vi "subGetItemInfosFromProjectFile.vi"(8 "error in (no error)":errorcluster, 11 "SolutionBuilder in":refnum<class "SolutionBuilder.lvclass">) -> (0 "error out":errorcluster, 3 "SolutionBuilder out":refnum<class "SolutionBuilder.lvclass">)   [LabVIEW 2019, in "SolutionBuilder.lvlib" / "SolutionBuilder.lvclass"]
uses:
  SolutionBuilder.lvclass
  SolutionBuilder.lvclass/SolutionBuilder.ctl
  ProjectItem/ProjectItem.lvclass
  ProjectItem/ProjectItem.lvclass/ProjectItem.ctl
  1413a22b-f5ab-415a-875b-e08797a96725.vi
  <vilib>/xml/Load XML File.vi
  <vilib>/xml/Close Reference(Node).vi
  <vilib>/xml/NI_XML.lvlib
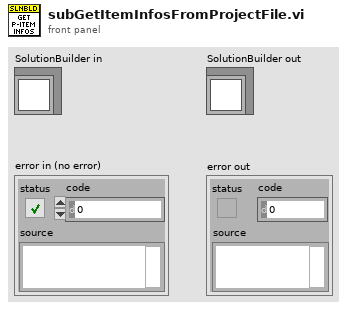
[diagram p1: front panel]
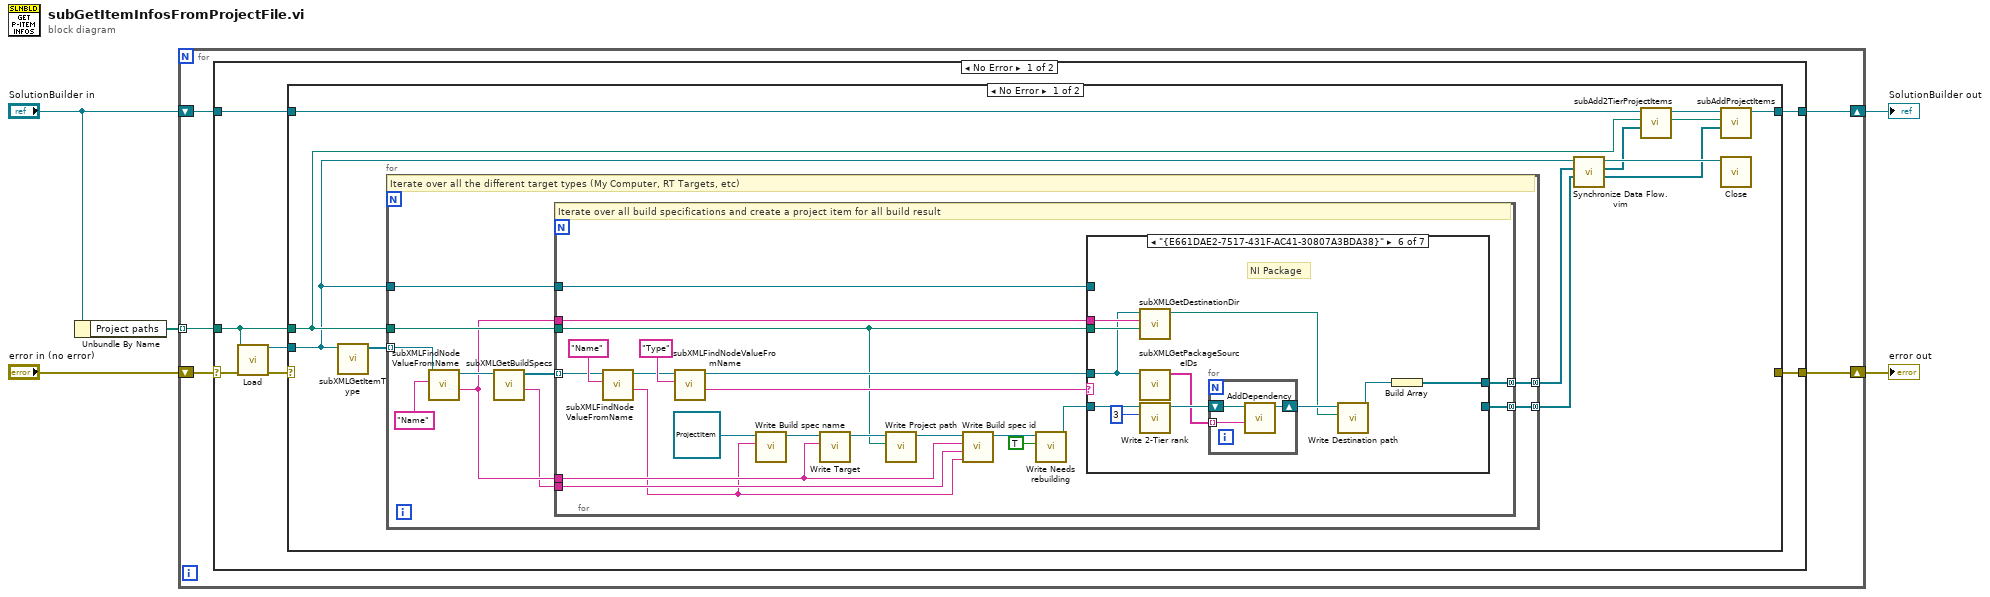
[diagram p0: block diagram]
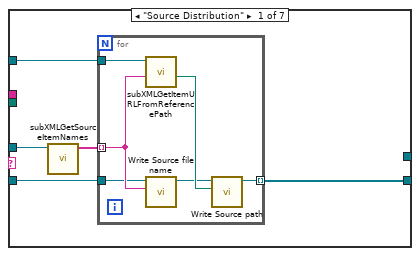
[diagram p2: hidden frame]
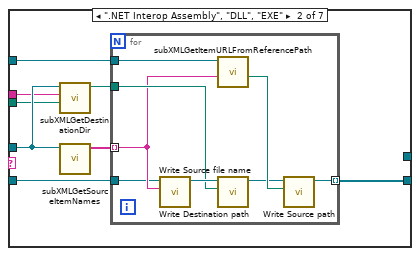
[diagram p3: hidden frame]
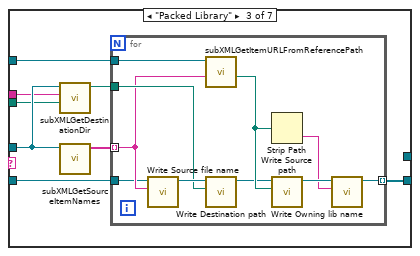
[diagram p4: hidden frame]
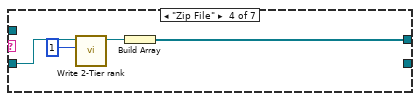
[diagram p5: hidden frame]
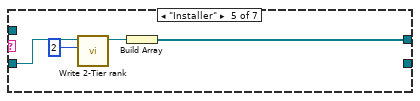
[diagram p6: hidden frame]
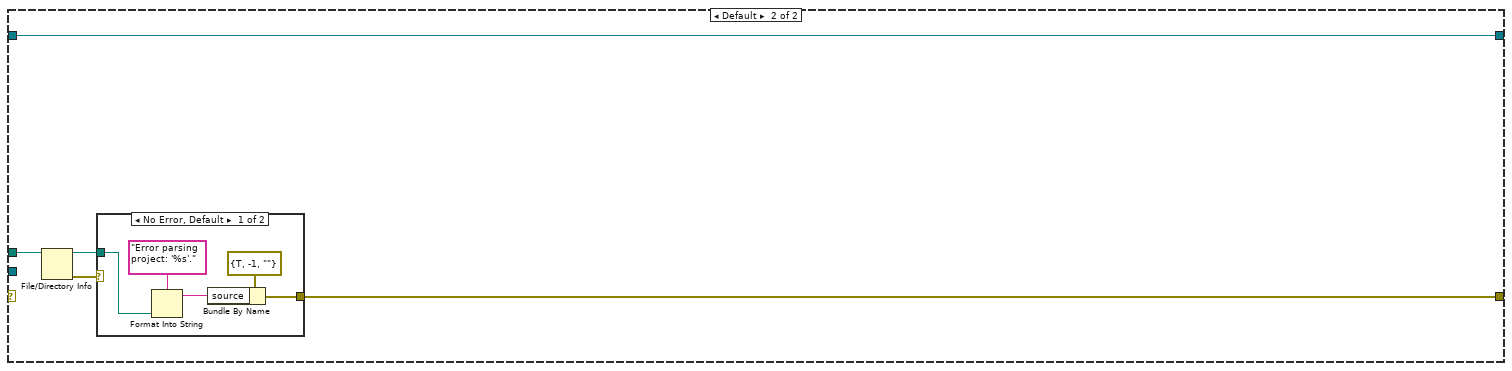
[diagram p8: hidden frame]
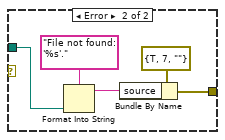
[diagram p9: hidden frame]
diagram:
  n1 = Unbundle By Name("SolutionBuilder in") -> ("Project paths"=w5:path[])
  n2 = for {
    tunnel: w5 -> [w9] mode=indexing
    shift-right: [w8] -> w3
    shift-left: "SolutionBuilder in" -> [w10]
    shift-right: [w7] -> w2
    shift-left: "error in (no error)" -> [w6]
    n3 = case shown="No Error" w6 {
      selector: w6 -> [w11 w143]
      tunnel: w10 -> [w16 w142]
      tunnel: w9 -> [w15 _]
      tunnel: [w14 w142] -> w8
      tunnel: [w12 w143] -> w7
      frame No Error {
        n4 = call-poly <vilib>:"Load.vi"("path to XML document"=w15, "error in (no error)"=w11) -> ("DOM document out"=w17:refnum<k20>, "error out"=w13:errorcluster)  [unwired: 11 in, 1 out]
        n5 = case shown="No Error" w13 {
          tunnel: w17 -> [w21 _]
          tunnel: w16 -> [w25 w131]
          tunnel: w15 -> [w23 w128]
          tunnel: [w28 w131] -> w14
          tunnel: [_ w130] -> w12
          frame No Error {
            n6 = call "subXMLGetItemType.vi"("Refnum in"=w21) -> ("Nodes"=w20:refnum<k20>[])  [unwired: 10 in]
            n7 = for {
              tunnel: [w37] -> w19 mode=concatenating
              tunnel: [w36] -> w18 mode=concatenating
              tunnel: w23 -> [w35]
              tunnel: w21 -> [w34]
              tunnel: w20 -> [w32] mode=indexing
              # "Iterate over all the different target types (My Computer, RT Targets, etc)"
              n8 = call "subXMLFindNodeValueFromName.vi"("Property name"="Name", "Refnum in"=w32) -> ("Value"=w30:string, "Refnum out"=w31:refnum<k20>)  [unwired: 7 in, 1 out]
              n9 = call "subXMLGetBuildSpecs.vi"("Refnum in"=w31) -> ("Buid spec section"=w29:string, "Nodes"=w38:refnum<k20>[])  [unwired: 9 in]
              n10 = for {
                tunnel: w38 -> [w54] mode=indexing
                tunnel: w35 -> [w44]
                tunnel: [w53] -> w37 mode=concatenating
                tunnel: w34 -> [w52]
                tunnel: [w51] -> w36 mode=concatenating
                tunnel: w30 -> [w40]
                tunnel: w30 -> [w50]
                tunnel: w29 -> [w45]
                # "Iterate over all build specifications and create a project item for all build result"
                n11 = call "subXMLFindNodeValueFromName.vi"("Property name"="Name", "Refnum in"=w54) -> ("Value"=w39:string, "Refnum out"=w55:refnum<k20>)  [unwired: 7 in, 1 out]
                n12 = call "subXMLFindNodeValueFromName.vi"("Property name"="Type", "Refnum in"=w55) -> ("Value"=w58:string, "Refnum out"=w57:refnum<k20>)  [unwired: 7 in, 1 out]
                n13 = call "Write Build spec name.vi"("Build spec name"=w39, "ProjectItem in"=refnum<class "ProjectItem.lvclass"> refnum ("SolutionBuilder.lvlib:ProjectItem.lvclass")) -> ("ProjectItem out"=w48:refnum<class "ProjectItem.lvclass">)  [unwired: 9 in]
                n14 = call "Write Target.vi"("Target"=w40, "ProjectItem in"=w48) -> ("ProjectItem out"=w49:refnum<class "ProjectItem.lvclass">)  [unwired: 9 in]
                n15 = call "Write Project path.vi"("Project path"=w44, "ProjectItem in"=w49) -> ("ProjectItem out"=w46:refnum<class "ProjectItem.lvclass">)  [unwired: 9 in]
                n16 = call-dynamic "Write Build spec id.vi"("Build spec name"=w39, "Buid spec section"=w45, "Target"=w40, "ProjectItem in"=w46) -> ("ProjectItem out"=w42:refnum<class "ProjectItem.lvclass">)  [unwired: 7 in]
                n17 = call "Write Needs rebuilding.vi"("Needs rebuilding"=TRUE, "ProjectItem in"=w42) -> ("ProjectItem out"=w41:refnum<class "ProjectItem.lvclass">)  [unwired: 9 in]
                n18 = case shown="\"{E661DAE2-7517-431F-AC41-30807A3BDA38}\"" w58 {
                  tunnel: w57 -> [w64 w76 w92 _ _ w113 _]
                  tunnel: [w62 w77 w93 _ _ _ _] -> w53
                  tunnel: w52 -> [w61 w74 w90 _ _ _ _]
                  tunnel: [_ _ _ w106 w110 w122 _] -> w51
                  tunnel: w50 -> [_ w73 w89 _ _ w118 _]
                  tunnel: w41 -> [w60 w72 w88 w105 w109 w121 _]
                  tunnel: w44 -> [_ w71 w87 _ _ w117 _]
                  frame "Source Distribution" {
                    n19 = call "subXMLGetSourceItemNames.vi"("Refnum in"=w64) -> ("Names"=w63:string[])  [unwired: 10 in]
                    n20 = for {
                      tunnel: w63 -> [w69] mode=indexing
                      tunnel: [w67] -> w62 mode=indexing
                      tunnel: w61 -> [w70]
                      tunnel: w60 -> [w65]
                      n21 = call "subXMLGetItemURLFromReferencePath.vi"("Reference path"=w69, "Root ref"=w70) -> ("Path"=w68:path)  [unwired: 7 in, 2 out]
                      n22 = call "Write Source file name.vi"("Source file name"=w69, "ProjectItem in"=w65) -> ("ProjectItem out"=w66:refnum<class "ProjectItem.lvclass">)  [unwired: 9 in]
                      n23 = call "Write Source path.vi"("Source path"=w68, "ProjectItem in"=w66) -> ("ProjectItem out"=w67:refnum<class "ProjectItem.lvclass">)  [unwired: 9 in]
                    }
                  }
                  frame ".NET Interop Assembly", "DLL", "EXE" {
                    n24 = call "subXMLGetDestinationDir.vi"("Project path"=w71, "TargetName"=w73, "Refnum in"=w76) -> ("Path"=w75:path)  [unwired: 7 in, 1 out]
                    n25 = call "subXMLGetSourceItemNames.vi"("Refnum in"=w76) -> ("Names"=w78:string[])  [unwired: 10 in]
                    n26 = for {
                      tunnel: w78 -> [w83] mode=indexing
                      tunnel: [w81] -> w77 mode=indexing
                      tunnel: w75 -> [w85]
                      tunnel: w74 -> [w84]
                      tunnel: w72 -> [w80]
                      n27 = call "Write Source file name.vi"("Source file name"=w83, "ProjectItem in"=w80) -> ("ProjectItem out"=w86:refnum<class "ProjectItem.lvclass">)  [unwired: 9 in]
                      n28 = call "subXMLGetItemURLFromReferencePath.vi"("Reference path"=w83, "Root ref"=w84) -> ("Path"=w82:path)  [unwired: 7 in, 2 out]
                      n29 = call "Write Destination path.vi"("Destination path"=w85, "ProjectItem in"=w86) -> ("ProjectItem out"=w79:refnum<class "ProjectItem.lvclass">)  [unwired: 9 in]
                      n30 = call "Write Source path.vi"("Source path"=w82, "ProjectItem in"=w79) -> ("ProjectItem out"=w81:refnum<class "ProjectItem.lvclass">)  [unwired: 9 in]
                    }
                  }
                  frame "Packed Library" {
                    n31 = call "subXMLGetDestinationDir.vi"("Project path"=w87, "TargetName"=w89, "Refnum in"=w92) -> ("Path"=w91:path)  [unwired: 7 in, 1 out]
                    n32 = call "subXMLGetSourceItemNames.vi"("Refnum in"=w92) -> ("Names"=w94:string[])  [unwired: 10 in]
                    n33 = for {
                      tunnel: w94 -> [w101] mode=indexing
                      tunnel: [w99] -> w93 mode=indexing
                      tunnel: w91 -> [w103]
                      tunnel: w90 -> [w102]
                      tunnel: w88 -> [w95]
                      n34 = call "Write Source file name.vi"("Source file name"=w101, "ProjectItem in"=w95) -> ("ProjectItem out"=w104:refnum<class "ProjectItem.lvclass">)  [unwired: 9 in]
                      n35 = call "subXMLGetItemURLFromReferencePath.vi"("Reference path"=w101, "Root ref"=w102) -> ("Path"=w98:path)  [unwired: 7 in, 2 out]
                      n36 = call "Write Destination path.vi"("Destination path"=w103, "ProjectItem in"=w104) -> ("ProjectItem out"=w96:refnum<class "ProjectItem.lvclass">)  [unwired: 9 in]
                      n37 = Strip Path(path=w98) -> (name=w97:string)  [unwired: 1 out]
                      n38 = call "Write Source path.vi"("Source path"=w98, "ProjectItem in"=w96) -> ("ProjectItem out"=w100:refnum<class "ProjectItem.lvclass">)  [unwired: 9 in]
                      n39 = call "Write Owning lib name.vi"("Owning lib name"=w97, "ProjectItem in"=w100) -> ("ProjectItem out"=w99:refnum<class "ProjectItem.lvclass">)  [unwired: 9 in]
                    }
                  }
                  frame "Zip File" {
                    n40 = call "Write 2-Tier rank.vi"("2-Tier rank"=u8 1, "ProjectItem in"=w105) -> ("ProjectItem out"=w108:refnum<class "ProjectItem.lvclass">)  [unwired: 9 in]
                    n41 = Build Array(w108) -> (w106:refnum<class "ProjectItem.lvclass">[])
                  }
                  frame "Installer" {
                    n42 = call "Write 2-Tier rank.vi"("2-Tier rank"=u8 2, "ProjectItem in"=w109) -> ("ProjectItem out"=w112:refnum<class "ProjectItem.lvclass">)  [unwired: 9 in]
                    n43 = Build Array(w112) -> (w110:refnum<class "ProjectItem.lvclass">[])
                  }
                  frame "{E661DAE2-7517-431F-AC41-30807A3BDA38}" {
                    # "NI Package"
                    n44 = call "subXMLGetDestinationDir.vi"("Project path"=w117, "TargetName"=w118, "Refnum in"=w113) -> ("Path"=w114:path)  [unwired: 7 in, 1 out]
                    n45 = call "subXMLGetPackageSourceIDs.vi"("Refnum in"=w113) -> ("IDs"=w119:string[])  [unwired: 10 in]
                    n46 = call "Write 2-Tier rank.vi"("2-Tier rank"=u8 3, "ProjectItem in"=w121) -> ("ProjectItem out"=w120:refnum<class "ProjectItem.lvclass">)  [unwired: 9 in]
                    n47 = for {
                      shift-right: [w125] -> w116
                      shift-left: w120 -> [w126]
                      tunnel: w119 -> [w124] mode=indexing
                      n48 = call "AddDependency.vi"("Dependency"=w124, "ProjectItem in"=w126) -> ("ProjectItem out"=w125:refnum<class "ProjectItem.lvclass">)  [unwired: 8 in, 1 out]
                    }
                    n49 = call "Write Destination path.vi"("Destination path"=w114, "ProjectItem in"=w116) -> ("ProjectItem out"=w115:refnum<class "ProjectItem.lvclass">)  [unwired: 9 in]
                    n50 = Build Array(w115) -> (w122:refnum<class "ProjectItem.lvclass">[])
                  }
                  frame Default {
                  }
                }
              }
            }
            n51 = call "Synchronize Data Flow.vim"("input 3"=w19, "input 2"=w18, "input 1"=w21) -> ("output 3"=w26:refnum<class "ProjectItem.lvclass">[], "output 2"=w22:refnum<class "ProjectItem.lvclass">[], "output 1"=w27:refnum<k20>)  [unwired: 1 in, 1 out]
            n52 = call "subAdd2TierProjectItems.vi"("ProjectItems"=w22, "Owning project"=w23, "SolutionBuilder in"=w25) -> ("SolutionBuilder out"=w24:refnum<class "SolutionBuilder.lvclass">)  [unwired: 7 in, 1 out]
            n53 = call "subAddProjectItems.vi"("ProjectItems"=w26, "Owning project"=w23, "SolutionBuilder in"=w24) -> ("SolutionBuilder out"=w28:refnum<class "SolutionBuilder.lvclass">)  [unwired: 7 in, 1 out]
            n54 = call-poly <vilib>:"Close.vi"("node"=w27) -> ()  [unwired: 8 in, 1 out]
          }
          frame Default {
            n55 = File/Directory Info(path=w128) -> (path out=w129:path, error out=w127:errorcluster)  [unwired: 1 in, 5 out]
            n56 = case shown="No Error, Default" w127 {
              tunnel: [w133 w138] -> w130
              tunnel: w129 -> [w132 w137]
              frame No Error {
                n57 = Format Into String(format string="Error parsing project: '%s'.", w132) -> (resulting string=w135:string)  [unwired: 2 in, 1 out]
                n58 = Bundle By Name(cluster=errorcluster {"status"=TRUE, "code"=-1, "source"=""} ("t"), "source"=w135) -> (w133:errorcluster)
              }
              frame Error {
                n59 = Format Into String(format string="File not found: '%s'.", w137) -> (resulting string=w140:string)  [unwired: 2 in, 1 out]
                n60 = Bundle By Name(cluster=errorcluster {"status"=TRUE, "code"=7, "source"=""} ("t"), "source"=w140) -> (w138:errorcluster)
              }
            }
          }
        }
      }
      frame Error {
      }
    }
  }
  "SolutionBuilder out" <- w3
  "error out" <- w2
